vi "SMTP Email Keyed Array Add.vi"(4 "case matching (sensitive)":T1=enum."system", 5 "value":string, 6 "key":string, 7 "array in":T2) -> (1 "replaced":bool, 2 "prev value":string, 3 "array out":T2)   [LabVIEW 2011, in "NewNI_SMTPEmail.lvlib"]
uses:
  NewNI_SMTPEmail.lvlib
  SMTP Email Keyed Array.ctl
  SMTP Email Case Matching.ctl
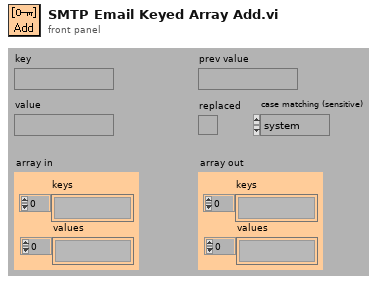
[diagram p1: front panel]
types:
  T1 = typedef "NewNI_SMTPEmail.lvlib/SMTP Email Case Matching.ctl" = enum16{"a != A", "a == A", "system"}
  T2 = typedef "NewNI_SMTPEmail.lvlib/SMTP Email Keyed Array.ctl" = cluster{"keys":string[], "values":string[]}
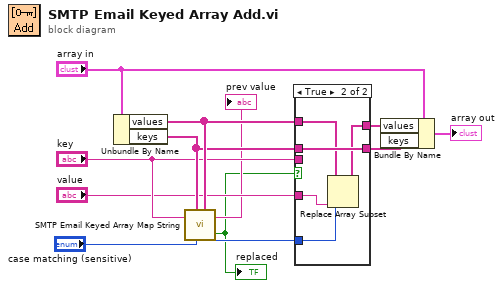
[diagram p0: block diagram]
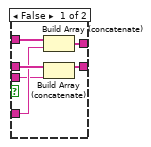
[diagram p2: hidden frame]
diagram:
  n1 = Unbundle By Name("array in") -> ("values"=w8:string[], "keys"=w7:string[])
  n2 = call "SMTP Email Keyed Array Map String.vi"("case matching (sensitive)"="case matching (sensitive)", "key"="key", "keys"=w7, "values"=w8) -> ("index"=w4:i32, "valid key"=w2:bool, "value"=→"prev value":string)  [unwired: 1 in]
  "replaced" <- w2
  n3 = case shown="True" w2 {
    tunnel: "value" -> [w14 w20]
    tunnel: "key" -> [w13 _]
    tunnel: w7 -> [w18 w23]
    tunnel: w8 -> [w17 w22]
    tunnel: [w16 w23] -> w9
    tunnel: [w15 w21] -> w10
    tunnel: w4 -> [_ w19]
    frame False {
      n4 = Build Array (concatenate)(w17, w14) -> (w15:string[])
      n5 = Build Array (concatenate)(w18, w13) -> (w16:string[])
    }
    frame True {
      n6 = Replace Array Subset(array=w22, new element=w20, index=w19) -> (w21:string[])
    }
  }
  n7 = Bundle By Name(cluster="array in", "values"=w10, "keys"=w9) -> (→"array out":T2)
